vi "Calls to random DQMH Modules for testing.vi"   [LabVIEW 2020]
uses:
  DQMH-Training/LabVIEW Code/Coins/Coins.lvlib
  DQMH-Training/LabVIEW Code/Products/Products.lvlib
  DQMH-Training/LabVIEW Code/UI Controller/UI Controller.lvlib
  <vilib>/PantherLAB/IMAQdx Camera/PantherLAB_lib_IMAQdx_CameraCamera.lvlib
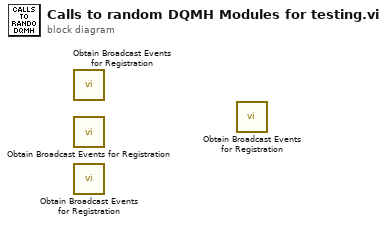
[diagram p0: block diagram]
diagram:
  n1 = call <vilib>:"Obtain Broadcast Events for Registration.vi"() -> ()  [unwired: 9 in, 3 out]
  n2 = call <vilib>:"Obtain Broadcast Events for Registration.vi"() -> ()  [unwired: 9 in, 3 out]
  n3 = call <vilib>:"Obtain Broadcast Events for Registration.vi"() -> ()  [unwired: 9 in, 3 out]
  n4 = call <vilib>:"Obtain Broadcast Events for Registration.vi"() -> ()  [unwired: 9 in, 3 out]
